vi "Find Minimum Indexes.vi"(10 "broken streaks":u8[](array[numeric]), 11 "map":i8[](array[numeric])) -> (3 "minimum indexes":u8[](array[numeric]))   [LabVIEW 2022 SP3]
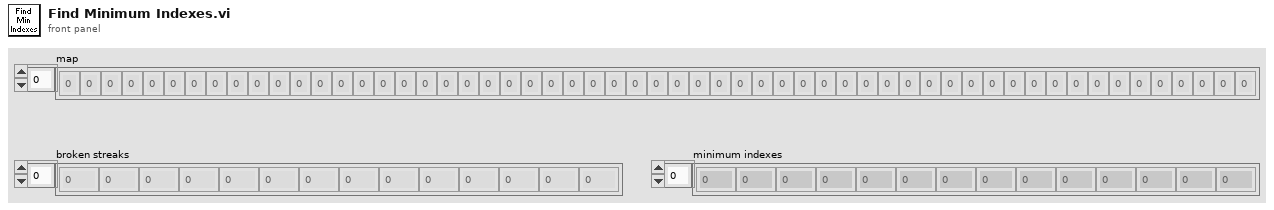
[diagram p1: front panel]
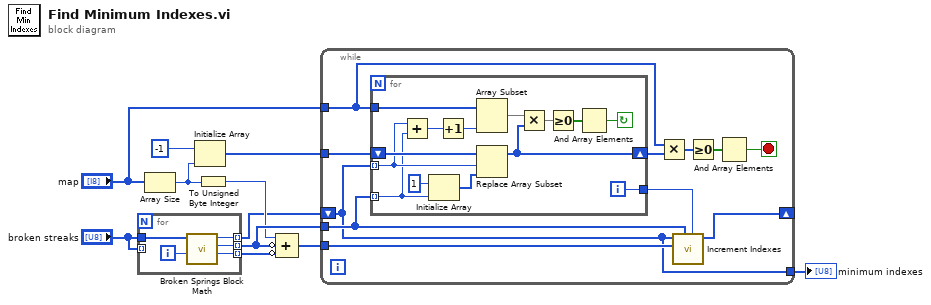
[diagram p0: block diagram]
diagram:
  n1 = for {
    tunnel: "broken streaks" -> [w16]
    tunnel: [w14] -> w2 mode=indexing
    tunnel: [w13] -> w7 mode=indexing
    tunnel: [w12] -> w1 mode=indexing
    tunnel: "broken streaks" -> [_] mode=indexing
    i -> [w15]
    n2 = call "Broken Springs Block Math.vi"("index"=w15, "contiguous length of broken springs"=w16) -> ("right total"=w12:u8, "current index broken streak length"=w13:u8, "left total"=w14:u8)  [unwired: 7 in]
  }
  n3 = Array Size(array="map") -> (size(s)=w4:i32)
  n4 = Initialize Array(i8 -1 ("unsigned 8bit integer"), w4) -> (w8:i8[])
  n5 = To Unsigned Byte Integer(number=w4) -> (unsigned 8bit integer=w5:u8)
  n6 = Compound Arithmetic op=ADD(w5, invert w7, invert w1) -> (w6:u8[])
  n7 = while {
    tunnel: w8 -> [w27]
    tunnel: w7 -> [w24]
    shift-right: [w25] -> _
    shift-left: w2 -> [w22]
    tunnel: w6 -> [w26]
    tunnel: "map" -> [w17]
    tunnel: [w22] -> w9
    stop <- w18 stop-if-true
    n8 = for {
      tunnel: w24 -> [w36] mode=indexing
      shift-right: [w33] -> w19
      shift-left: w27 -> [w41]
      tunnel: w22 -> [w37] mode=indexing
      tunnel: w17 -> [w38]
      tunnel: [w31] -> w23
      i -> [w31]
      stop <- w29 continue-if-true
      n9 = Add(x=w37, y=w36) -> (x+y=w35:u8)
      n10 = Initialize Array(i8 1 ("unsigned 8bit integer"), w36) -> (w40:i8[])
      n11 = Increment(x=w35) -> (x+1=w28:u8)
      n12 = Array Subset(array=w38, length=w28) -> (w34:i8[])  [unwired: 1 in]
      n13 = Replace Array Subset(array=w41, new element=w40, index=w37) -> (w33:i8[])
      n14 = Multiply(x=w34, y=w33) -> (x*y=w30:i8[])
      n15 = Greater Or Equal To 0?(x=w30) -> (x >= 0?=w32:bool[])
      n16 = And Array Elements(Boolean array=w32) -> (logical AND=w29:bool)
    }
    n17 = Multiply(x=w17, y=w19) -> (x*y=w20:i8[])
    n18 = call "Increment Indexes.vi"("group index to increment"=w23, "lengths"=w24, "max indexes"=w26, "previous indexes"=w22) -> ("next indexes"=w25:u8[])  [unwired: 5 in, 2 out]
    n19 = Greater Or Equal To 0?(x=w20) -> (x >= 0?=w21:bool[])
    n20 = And Array Elements(Boolean array=w21) -> (logical AND=w18:bool)
  }
  "minimum indexes" <- w9
